vi "Timestamp to Strings.vi"(6 "Input Time":timestamp) -> (0 "Filename Date":string, 1 "Filename Date-Time":string, 2 "DB Date-Time":string, 3 "Unique ID":string)   [LabVIEW 2010]
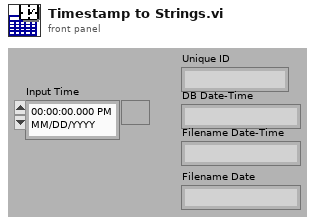
[diagram p1: front panel]
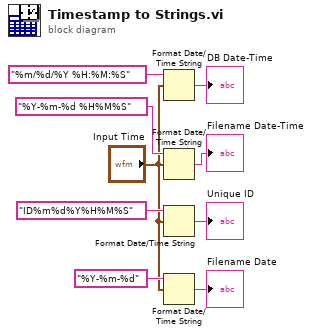
[diagram p0: block diagram]
diagram:
  n1 = Format Date/Time String(time format string (%c)="%m/%d/%Y %H:%M:%S", seconds (now)="Input Time") -> (date/time string=→"DB Date-Time":string)  [unwired: 1 in]
  n2 = Format Date/Time String(time format string (%c)="%Y-%m-%d %H%M%S", seconds (now)="Input Time") -> (date/time string=→"Filename Date-Time":string)  [unwired: 1 in]
  n3 = Format Date/Time String(time format string (%c)="ID%m%d%Y%H%M%S", seconds (now)="Input Time") -> (date/time string=→"Unique ID":string)  [unwired: 1 in]
  n4 = Format Date/Time String(time format string (%c)="%Y-%m-%d", seconds (now)="Input Time") -> (date/time string=→"Filename Date":string)  [unwired: 1 in]
